vi "DepthSense Demo.vi"() -> ()   [LabVIEW 2011]
panel:
  in  "stop 2":bool
  out "Image 2":T1(plugin-control)
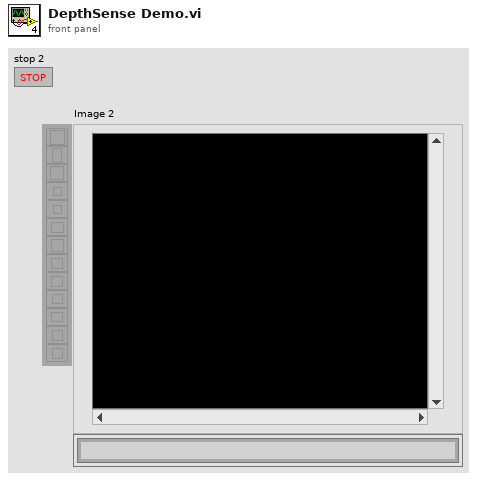
[diagram p1: front panel]
types:
  T1 = typedef "IMAQ Image.ctl" = refnum<image>
  T2 = typedef "t_CallbackReferences.ctl" = cluster{"LV event callback ":refnum<k27>, "Proxy instance":refnum<k24>, "(*f)(...)":i32}
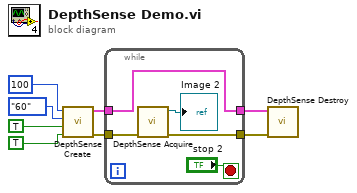
[diagram p0: block diagram]
diagram:
  n1 = call "DepthSense Create.vi"("Denoise?"=TRUE, "Close Mode?"=TRUE, "Framerate"=enum32{"25", "30", "50", "60"}."60", "Confidence"=100) -> ("error out"=w8:errorcluster, "callbacks"=w6:cluster{"References":T2, "References":T2})  [unwired: 5 in, 1 out]
  n2 = while {
    tunnel: w8 -> [w13]
    tunnel: [w11] -> w7
    tunnel: [w10] -> w5
    tunnel: w6 -> [w10]
    stop <- "stop 2" stop-if-true
    n3 = call "DepthSense Acquire.vi"("error in (no error)"=w13) -> ("error out"=w11:errorcluster, "new depth frame"=→"Image 2":T1)  [unwired: 9 in]
  }
  n4 = call "DepthSense Destroy.vi"("error in (no error)"=w7, "callbacks"=w5) -> ()  [unwired: 10 in]
